vi "Match subrate.vi"(10 "regular expression":string, 11 "data string 3":string) -> (2 "After":string, 3 "Before":string)   [LabVIEW 2020]
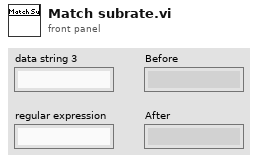
[diagram p1: front panel]
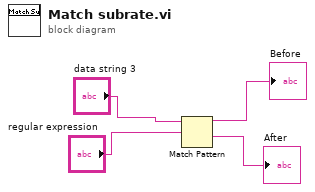
[diagram p0: block diagram]
diagram:
  n1 = Match Pattern(string="data string 3", regular expression="regular expression") -> (before substring=→"Before":string, after substring=→"After":string)  [unwired: 1 in, 2 out]
